vi "Fetch.vi"(8 "error in":errorcluster, 10 "Fetch Type":i32(ring) items=["Current", "Power", "Voltage", "Capacity", "Time"], 11 "VISA resource name":refnum<visa-resource-name>) -> (0 "error out":errorcluster, 2 "Value":dbl, 3 "VISA resource name out":refnum<visa-resource-name>)   [LabVIEW 2018, in "IT-M3100.lvlib"]
doc: "The command to get the following average.\n<b>Fetch Type</b>\n0:Current:Return the current average of measurements.\n1:Power:Return to measure the power of the average.\n2:Voltage:Average return to measure the voltage.\n3:Capacity:Returns the capacity of battery charging and discharging.\n4:Time:Returns the time timer."
uses:
  IT-M3100.lvlib
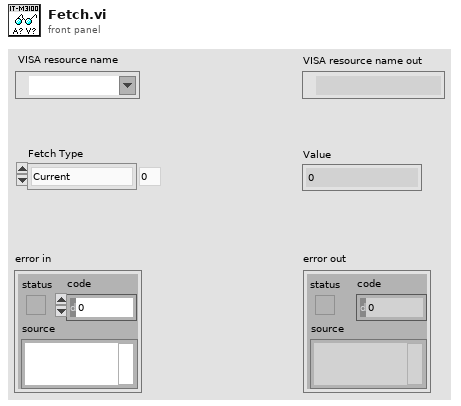
[diagram p1: front panel]
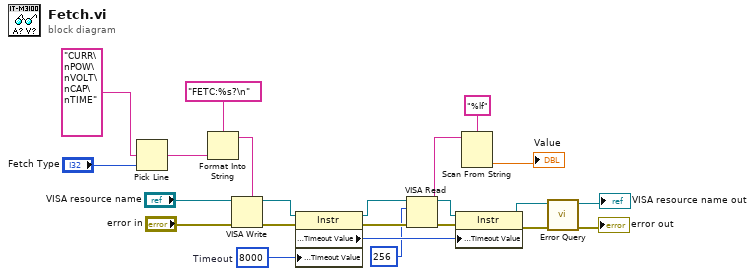
[diagram p0: block diagram]
diagram:
  w21 = u32 8000  # Timeout
  n1 = Pick Line(multi-line string="CURR\nPOW\nVOLT\nCAP\nTIME", line index="Fetch Type") -> (output string=w8:string)  [unwired: 1 in]
  n2 = Format Into String(format string="FETC:%s?\n", w8) -> (resulting string=w11:string)  [unwired: 2 in, 1 out]
  n3 = VISA Write(VISA resource name="VISA resource name", write buffer=w11, error in (no error)="error in") -> (VISA resource name out=w23:refnum<visa-resource-name>, error out=w22:errorcluster)  [unwired: 1 out]
  n4 = property class="Instr"(reference=w23, error in=w22, "General Settings:Timeout Value"=w21) -> (reference out=w16:refnum<visa-resource-name>, error out=w17:errorcluster, "General Settings:Timeout Value"=w18:u32)
  n5 = VISA Read(VISA resource name=w16, byte count=256, error in (no error)=w17) -> (VISA resource name out=w20:refnum<visa-resource-name>, read buffer=w13:string, error out=w19:errorcluster)  [unwired: 1 out]
  n6 = property class="Instr"(reference=w20, error in=w19, "General Settings:Timeout Value"=w18) -> (reference out=w1:refnum<visa-resource-name>, error out=w2:errorcluster)
  n7 = Scan From String(format string="%lf", input string=w13) -> (output 1=→"Value":dbl)  [unwired: 3 in, 3 out]
  n8 = call "Error Query.vi"("error in"=w2, "VISA resource name"=w1) -> ("error out"=→"error out":errorcluster, "VISA resource name out"=→"VISA resource name out":refnum<visa-resource-name>)  [unwired: 6 in, 2 out]
